vi "top_close_devices.vi"(8 "error in (no error)":errorcluster, 9 "Front_panel_refs":T1, 10 "Dynamic data":T2, 11 "Input parameters":T3={"Measurement type"=enum."Debug", "Sensor type"=enum."HPK_8in_271ch", "Identifier"="test.txt", "Open after execution?"=FALSE, "Plot after execution?"=FALSE, "Display channel"=0, "Voltage Delay (s)"=0.5, "Switch Delay (s)"=0.01, "VISA resource name source"="", "VISA resource name DMM"="", "VISA resource name LCR"="", "Compliance  Level (A)"=10.0, "Voltage Limit (V)"=1000.0, "Data storage location"="", "Scan voltages"="", "Use source as DMM?"=FALSE, "LCR signal frequenzy (Hz)"=10.0, "DMM device"=enum."Keithley2001", "Sampling number"=1, "Use env. sensors on"=enum."Sensirion sht1x/7x", "Switchboard Handle"=0, "Use Switchboard"=FALSE, "LCR signal voltage (V)"=10000.0, "Repeat"=1, "Scan voltages IV"="", "Scan voltages CV"="", "Hex pad numbers?"=FALSE, "Set measurement type"=enum."Debug", "Custom pad scan"="", "IV voltage Delay (s)"=0.5, "CV voltage Delay (s)"=0.5, "Needle measurement?"=FALSE, "Comments"="test.txt", "LCR signal frequenzy (kHz)"=10.0, "Compliance  Level (uA)"=10.0, "Open Correction Array"=array2304x3[6912 elements], "Current set voltage"=0.0, "Last set voltage"=0.0, "Current channel"=0, "Last OpenCorrection index"=-1, "Total curr/vltg every x steps"=10, "Current channel iteration"=0, "No CV corrections"=FALSE, "Mapfile"="", "Corrfile"="", "IV voltage file"=path "", "CV voltage file"=path "", "IV Switch Delay (s)"=0.01, "CV Switch Delay (s)"=0.01, "Invert polarity"=FALSE, "Set debug dirs"=FALSE, "Is n on p"=FALSE, "Source interlock?"=TRUE, "Voltage file used?"=FALSE, "Pad mask"="", "Mask pad above (uA)"=1.0, "LCR device"=enum."LCR_E4980", "Source device"=enum."Source_2410", "HexPlot binary path"="", "PadReductionFactor"=1.0, "Temperature degC"="", "Fluence [neq]"="", "Annealing [min]"=""} {"CV Switch Delay (s)" format="%#_13g"; "IV Switch Delay (s)" format="%#_13g"; "Last set voltage" format="%#_13g"; "Current set voltage" format="%#_13g"; "CV voltage Delay (s)" format="%#_13g"; "IV voltage Delay (s)" format="%#_13g"; "Voltage Limit (V)" format="%#_13g"; "Voltage Delay (s)" format="%#_13g"; "Switch Delay (s)" format="%#_13g"}) -> (0 "error out":errorcluster, 1 "Front_panel_refs out":T1, 2 "Dynamic data":T2, 3 "Input parameters":T3={"Measurement type"=enum."Debug", "Sensor type"=enum."HPK_8in_271ch", "Identifier"="test.txt", "Open after execution?"=FALSE, "Plot after execution?"=FALSE, "Display channel"=0, "Voltage Delay (s)"=0.5, "Switch Delay (s)"=0.01, "VISA resource name source"="", "VISA resource name DMM"="", "VISA resource name LCR"="", "Compliance  Level (A)"=10.0, "Voltage Limit (V)"=1000.0, "Data storage location"="", "Scan voltages"="", "Use source as DMM?"=FALSE, "LCR signal frequenzy (Hz)"=10.0, "DMM device"=enum."Keithley2001", "Sampling number"=1, "Use env. sensors on"=enum."Sensirion sht1x/7x", "Switchboard Handle"=0, "Use Switchboard"=FALSE, "LCR signal voltage (V)"=10000.0, "Repeat"=1, "Scan voltages IV"="", "Scan voltages CV"="", "Hex pad numbers?"=FALSE, "Set measurement type"=enum."Debug", "Custom pad scan"="", "IV voltage Delay (s)"=0.5, "CV voltage Delay (s)"=0.5, "Needle measurement?"=FALSE, "Comments"="test.txt", "LCR signal frequenzy (kHz)"=10.0, "Compliance  Level (uA)"=10.0, "Open Correction Array"=array2304x3[6912 elements], "Current set voltage"=0.0, "Last set voltage"=0.0, "Current channel"=0, "Last OpenCorrection index"=-1, "Total curr/vltg every x steps"=10, "Current channel iteration"=0, "No CV corrections"=FALSE, "Mapfile"="", "Corrfile"="", "IV voltage file"=path "", "CV voltage file"=path "", "IV Switch Delay (s)"=0.01, "CV Switch Delay (s)"=0.01, "Invert polarity"=FALSE, "Set debug dirs"=FALSE, "Is n on p"=FALSE, "Source interlock?"=TRUE, "Voltage file used?"=FALSE, "Pad mask"="", "Mask pad above (uA)"=1.0, "LCR device"=enum."LCR_E4980", "Source device"=enum."Source_2410", "HexPlot binary path"="", "PadReductionFactor"=1.0, "Temperature degC"="", "Fluence [neq]"="", "Annealing [min]"=""} {"CV Switch Delay (s)" format="%#_13g"; "IV Switch Delay (s)" format="%#_13g"; "Last set voltage" format="%#_13g"; "Current set voltage" format="%#_13g"; "CV voltage Delay (s)" format="%#_13g"; "IV voltage Delay (s)" format="%#_13g"; "Voltage Limit (V)" format="%#_13g"; "Voltage Delay (s)" format="%#_13g"; "Switch Delay (s)" format="%#_13g"})   [LabVIEW 2020]
doc: "Closes the VISA connection to the instruments."
uses:
  input_params.ctl
  data_dynamic.ctl
  refs_front_panel.ctl
  <instrlib>/Keithley 24XX/Keithley 24XX.lvlib
  <instrlib>/Agilent 4263X/Agilent 4263X.lvlib
  <instrlib>/Agilent E4980/Agilent E4980.lvlib
  <instrlib>/Keithley 648X Series/Keithley 648X Series.lvlib
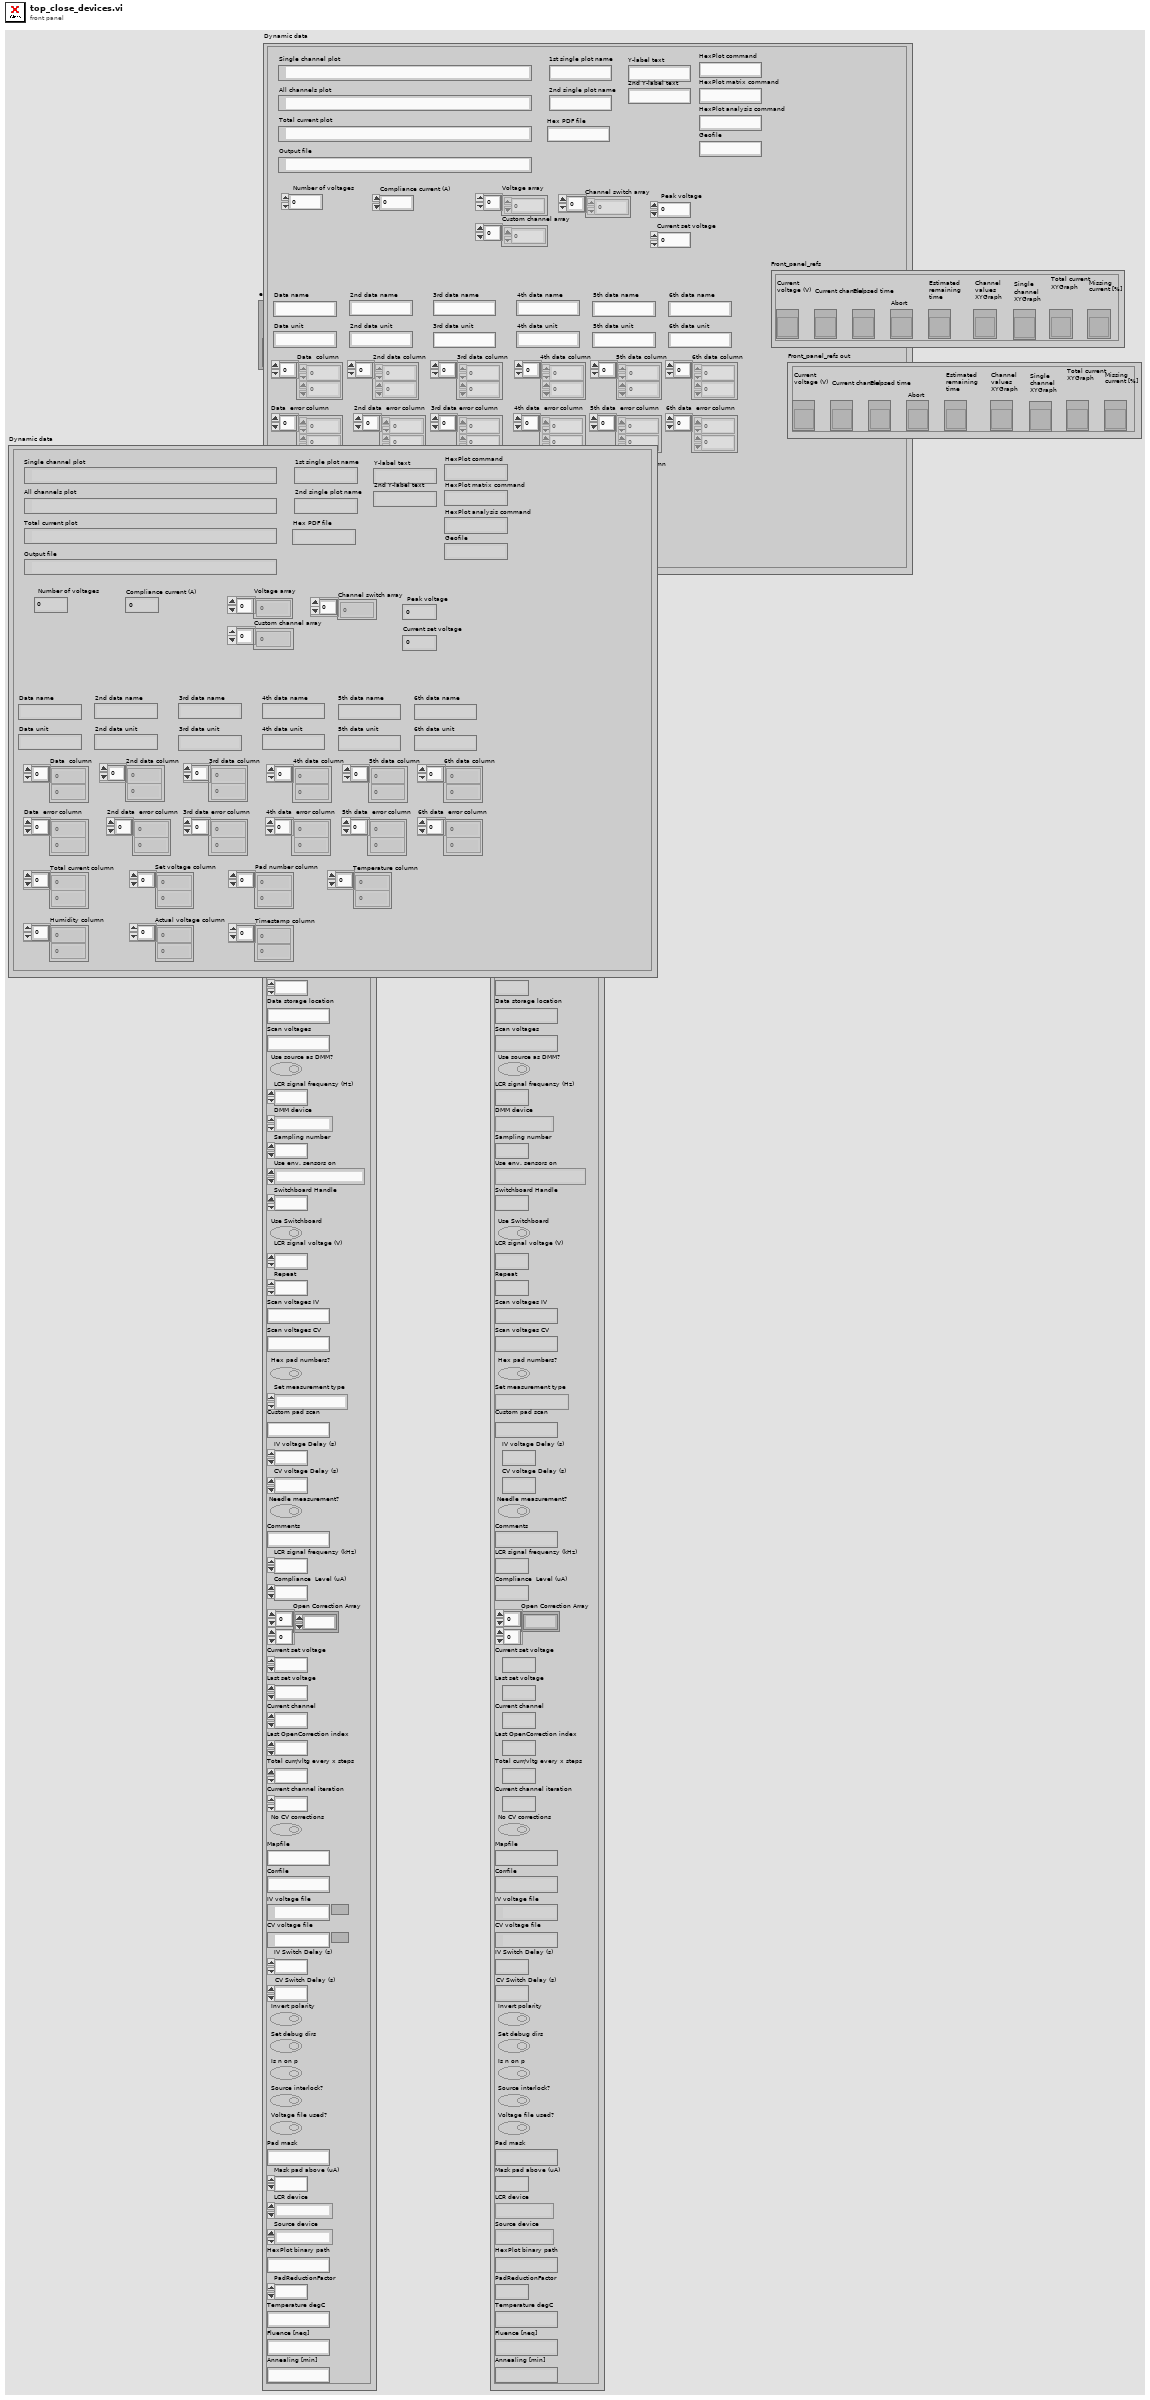
[diagram p1: front panel]
types:
  T1 = typedef "refs_front_panel.ctl" = cluster{"Current voltage (V)":refnum<vi>, "Elapsed time":refnum<vi>, "Current channel":refnum<vi>, "Abort":refnum<vi>, "Estimated remaining time":refnum<vi>, "Channel values XYGraph":refnum<vi>, "Single channel XYGraph":refnum<vi>, "Total current XYGraph":refnum<vi>, "Missing\ncurrent [%]":refnum<vi>}
  T2 = typedef "data_dynamic.ctl" = cluster{"Output file":path, "Y-label text":string, "Current set voltage":dbl, "Set voltage column":dbl[], "Pad number column":dbl[], "Data  column":dbl[], "Number of voltages":i32, "Compliance current (A)":dbl, "Geofile":string, "Peak voltage":dbl, "Hex PDF file":string, "Voltage array":dbl[], "Total current column":dbl[], "Timestamp column":dbl[], "Data name":string, "Data unit":string, "2nd data column":dbl[], "2nd data name":string, "2nd data unit":string, "3rd data column":dbl[], "4th data column":dbl[], "3rd data name":string, "3rd data unit":string, "4th data name":string, "4th data unit":string, "Actual voltage column":dbl[], "2nd Y-label text":string, "Single channel plot":path, "Temperature column":dbl[], "Humidity column":dbl[], "Channel switch array":i32[], "1st single plot name":string, "2nd single plot name":string, "All channels plot":path, "HexPlot command":string, "Custom channel array":i32[], "Data  error column":dbl[], "2nd data  error column":dbl[], "3rd data error column":dbl[], "4th data  error column":dbl[], "Total current plot":path, "5th data column":dbl[], "5th data  error column":dbl[], "6th data column":dbl[], "6th data  error column":dbl[], "5th data name":string, "5th data unit":string, "6th data name":string, "6th data unit":string, "HexPlot matrix command":string, "HexPlot analysis command":string}
  T3 = typedef "input_params.ctl" = cluster{"Measurement type":enum16{"IV", "CV", "Debug", "Test_contact"}, "Sensor type":enum16{"HPK_6in_135ch", "HPK_8in_271ch", "IFX_8in_256ch", "Diode", "HPK_6in_239ch", "Full_Matrix", "HPK_8in_271ch_full", "LumiCal", "HPK_8in_444ch", "HPK_8in_198ch_2019", "HPK_8in_MGW_LD_full", "HPK_8in_MGW_LD_a_type_top", "HPK_8in_MGW_LD_a_type_bottom", "HPK_8in_MGW_LD_b_type_left", "HPK_8in_MGW_LD_b_type_right", "HPK_8in_MGW_LD_c_type_left", "HPK_8in_MGW_LD_c_type_right", "HPK_8in_MGW_HD_full", "HPK_8in_MGW_HD_a_type_top", "HPK_8in_MGW_HD_a_type_bottom", "HPK_8in_MGW_HD_b_type_left", "HPK_8in_MGW_HD_b_type_right", "HPK_8in_MGW_HD_c_type_left", "HPK_8in_MGW_HD_c_type_right", "CALICE_6in_256ch"}, "Identifier":string, "Open after execution?":bool, "Plot after execution?":bool, "Display channel":i32, "Voltage Delay (s)":dbl, "Switch Delay (s)":dbl, "VISA resource name source":refnum<visa-resource-name>, "VISA resource name DMM":refnum<visa-resource-name>, "VISA resource name LCR":refnum<visa-resource-name>, "Compliance  Level (A)":dbl, "Voltage Limit (V)":dbl, "Data storage location":string, "Scan voltages":string, "Use source as DMM?":bool, "LCR signal frequenzy (Hz)":dbl, "DMM device":enum16{"Keithley2001", "Keithley2450", "Keithley2410", "Keithley6485", "Keithley6487", "Keithley6517"}, "Sampling number":i32, "Use env. sensors on":enum16{"Sensirion sht1x/7x", "Switch Matrix", "Probecard"}, "Switchboard Handle":u32, "Use Switchboard":bool, "LCR signal voltage (V)":dbl, "Repeat":i32, "Scan voltages IV":string, "Scan voltages CV":string, "Hex pad numbers?":bool, "Set measurement type":enum16{"IV", "CV", "Debug", "Test_contact", "IV+CV"}, "Custom pad scan":string, "IV voltage Delay (s)":dbl, "CV voltage Delay (s)":dbl, "Needle measurement?":bool, "Comments":string, "LCR signal frequenzy (kHz)":dbl, "Compliance  Level (uA)":dbl, "Open Correction Array":dbl[][], "Current set voltage":dbl, "Last set voltage":dbl, "Current channel":i32, "Last OpenCorrection index":i32, "Total curr/vltg every x steps":i32, "Current channel iteration":i32, "No CV corrections":bool, "Mapfile":string, "Corrfile":string, "IV voltage file":path, "CV voltage file":path, "IV Switch Delay (s)":dbl, "CV Switch Delay (s)":dbl, "Invert polarity":bool, "Set debug dirs":bool, "Is n on p":bool, "Source interlock?":bool, "Voltage file used?":bool, "Pad mask":string, "Mask pad above (uA)":dbl, "LCR device":enum16{"LCR_E4980", "AGILENT_4263X"}, "Source device":enum16{"Source_2410", "Source_6487"}, "HexPlot binary path":string, "PadReductionFactor":dbl, "Temperature degC":string, "Fluence [neq]":string, "Annealing [min]":string}
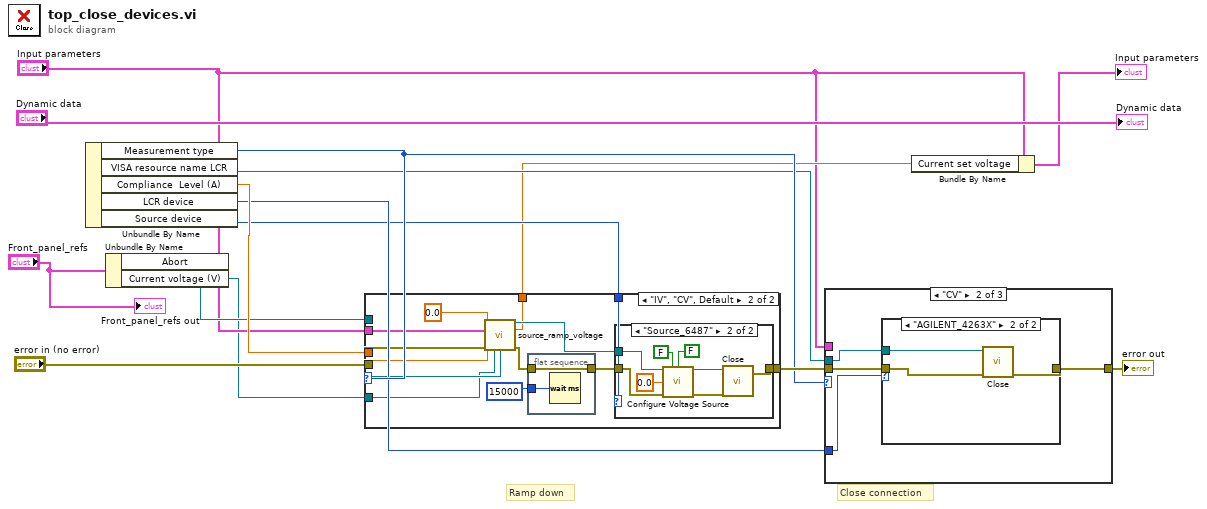
[diagram p0: block diagram]
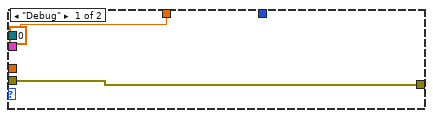
[diagram p2: hidden frame]
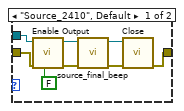
[diagram p3: hidden frame]
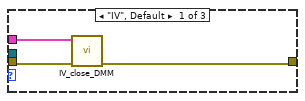
[diagram p4: hidden frame]
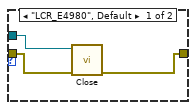
[diagram p5: hidden frame]
diagram:
  # "Close connection"
  # "Ramp down"
  n1 = Unbundle By Name("Input parameters") -> ("Measurement type"=w13:enum16{"IV", "CV", "Debug", "Test_contact"}, "VISA resource name LCR"=w11:refnum<visa-resource-name>, "Compliance  Level (A)"=w12:dbl, "LCR device"=w7:enum16{"LCR_E4980", "AGILENT_4263X"}, "Source device"=w6:enum16{"Source_2410", "Source_6487"})
  n2 = Unbundle By Name("Front_panel_refs") -> ("Abort"=w9:refnum<vi>, "Current voltage (V)"=w1:refnum<vi>)
  n3 = case shown="\"IV\", \"CV\", Default" w13 {
    tunnel: "error in (no error)" -> [w17 w30]
    tunnel: [w17 w28] -> w15
    tunnel: w12 -> [_ w29]
    tunnel: "Input parameters" -> [_ w27]
    tunnel: w9 -> [_ w26]
    tunnel: w6 -> [_ w21]
    tunnel: [0.0 ("Current voltage out (V)") w19] -> w5
    tunnel: w1 -> [_ w18]
    frame "Debug" {
    }
    frame "IV", "CV", Default {
      n4 = call "source_ramp_voltage.vi"("Input parameters"=w27, "Target voltage (V)"=0.0, "Compliance Current (A)"=w29, "error in (no error)"=w30, "Current source voltage reference"=w18, "Stop"=w26) -> ("VISA resource name out"=w22:refnum<visa-resource-name>, "Current voltage out (V)"=w19:dbl, "error out"=w24:errorcluster)  [unwired: 6 in, 1 out]
      n5 = flat-sequence {
        tunnel: u32 15000 ("milliseconds to wait") -> [w48]
        tunnel: w24 -> [w47]
        tunnel: [w47] -> w23
        frame #0 {
          n6 = Wait (ms)(milliseconds to wait=w48) -> ()  [unwired: 1 out]
        }
      }
      n7 = case shown="\"Source_6487\"" w21 {
        tunnel: [w33 w46] -> w28
        tunnel: w23 -> [w34 w43]
        tunnel: w22 -> [w32 w45]
        frame "Source_2410", Default {
          n8 = call <instrlib>:"Enable Output.vi"("error in (no error)"=w34, "Enable Output (T: Enable)"=FALSE ("Enable Output"), "VISA resource name"=w32) -> ("error out"=w35:errorcluster, "VISA resource name out"=w36:refnum<visa-resource-name>)  [unwired: 7 in]
          n9 = call "source_final_beep.vi"("error in (no error)"=w35, "VISA resource name"=w36) -> ("error out"=w38:errorcluster, "VISA resource name out"=w37:refnum<visa-resource-name>)  [unwired: 8 in]
          n10 = call <instrlib>:"Close.vi"("error in (no error)"=w38, "VISA resource name"=w37) -> ("error out"=w33:errorcluster)  [unwired: 9 in]
        }
        frame "Source_6487" {
          n11 = call <instrlib>:"Configure Voltage Source.vi"("VISA resource name"=w45, "Enable Voltage Source (F: Disable)"=FALSE, "Enable Interlock (F: Disable)"=FALSE, "Voltage Level (0 V)"=0.0, "error in (no error)"=w43) -> ("VISA resource name out"=w44:refnum<visa-resource-name>, "error out"=w42:errorcluster)  [unwired: 9 in]
          n12 = call <instrlib>:"Close.vi"("error in (no error)"=w42, "VISA resource name"=w44) -> ("error out"=w46:errorcluster)  [unwired: 9 in]
        }
      }
    }
  }
  n13 = case shown="\"CV\"" w13 {
    tunnel: w15 -> [w50 w55 w62]
    tunnel: [w51 w54 w62] -> w10
    tunnel: "Input parameters" -> [w49 _ _]
    tunnel: w11 -> [_ w53 _]
    tunnel: w7 -> [_ w52 _]
    frame "IV", Default {
      n14 = call "IV_close_DMM.vi"("error in (no error)"=w50, "Input parameters"=w49) -> ("error out"=w51:errorcluster)  [unwired: 9 in]
    }
    frame "CV" {
      n15 = case shown="\"AGILENT_4263X\"" w52 {
        tunnel: w55 -> [w57 w61]
        tunnel: [w56 w60] -> w54
        tunnel: w53 -> [w58 w59]
        frame "LCR_E4980", Default {
          n16 = call <instrlib>:"Close.vi"("error in (no error)"=w57, "VISA resource name"=w58) -> ("error out"=w56:errorcluster)  [unwired: 9 in]
        }
        frame "AGILENT_4263X" {
          n17 = call <instrlib>:"Close.vi"("error in (no error)"=w61, "VISA resource name"=w59) -> ("error out"=w60:errorcluster)  [unwired: 9 in]
        }
      }
    }
    frame "Debug" {
    }
  }
  "error out" <- w10
  n18 = Bundle By Name(cluster="Input parameters", "Current set voltage"=w5) -> (→"Input parameters":T3)
  "Dynamic data" <- "Dynamic data"
  "Front_panel_refs out" <- "Front_panel_refs"
